vi "mixed-lightsource-velleman.vi"(0 "Power Control":bool, 1 "Shutter VIS":bool, 2 "Shutter UV":bool, 3 "Select NKT System":enum32{"SuperK Varia (VIS)", "Extend-UV"}(radio), 4 "NKT Input Cluster":T2={"Power Level"=5.0, "Feedback Level"=0.0, "Short Wavelength (nm)"=560, "Long Wavelength (nm)"=580, "UV Wavelength (nm)"=400, "Emission On/Off"=FALSE, "Power/Feedback Mode"=FALSE} {"UV Wavelength (nm)" min=350 max=480 step=1; "Long Wavelength (nm)" min=501 max=850 step=1; "Short Wavelength (nm)" min=400 max=560 step=1; "Feedback Level" min=0.0 max=90.0 step=0.1 format="%.1f%%"; "Power Level" min=5.0 max=100.0 step=0.1 format="%.1f%%"}, 5 "Loop Count":i32, 14 "VISA in":refnum<visa-resource-name>, 15 "Init NKT?":bool) -> (6 "Shutter VIS":bool, 7 "Shutter UV 2":bool, 8 "Shutter UV":bool, 9 "Shutter VIS 2":bool, 10 "Laser On!":bool, 11 "Power Control 2":bool, 12 "NKT Output Cluster":T3 {"Feedback Level" format="%.1f%%"; "Power Level" format="%.1f%%"; "Temperature (°C)" format="%.1f"}, 13 "external control input changed?":bool, 17 "long wavelength":T1, 18 "short wavelength":T1, 19 "External Control Input Cluster":T2)   [LabVIEW 2015]
uses:
  <vilib>/Utility/miscctls.llb/LVMinMaxIncTypeDef.ctl
  PLEMv1/K8055D.dll
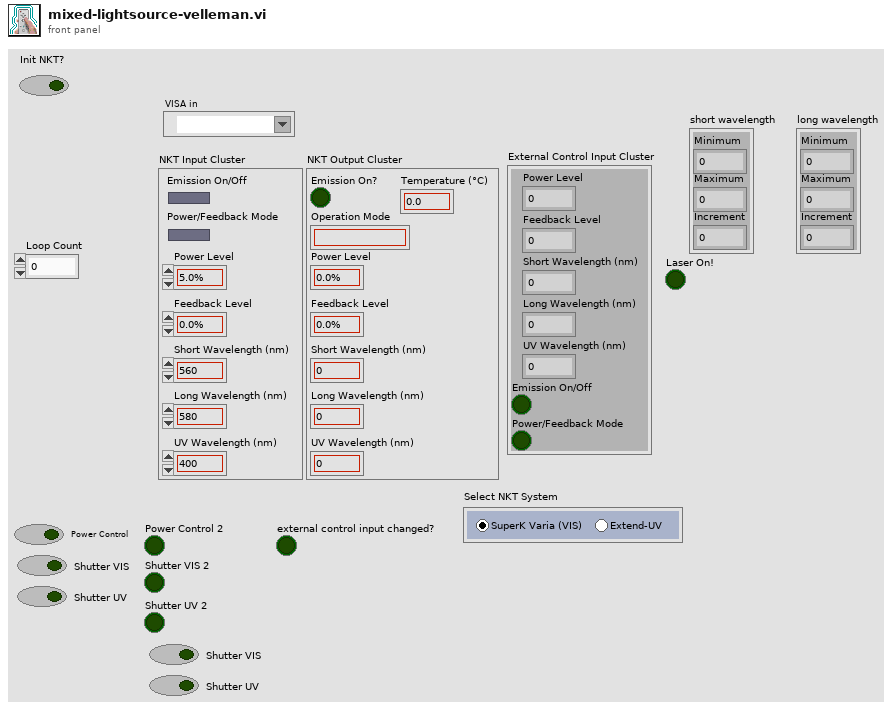
[diagram p1: front panel]
types:
  T1 = typedef "LVMinMaxIncTypeDef.ctl" = cluster{"Minimum":dbl, "Maximum":dbl, "Increment":dbl}
  T2 = cluster{"Power Level":dbl, "Feedback Level":dbl, "Short Wavelength (nm)":i32, "Long Wavelength (nm)":i32, "UV Wavelength (nm)":i32, "Emission On/Off":bool, "Power/Feedback Mode":bool}
  T3 = cluster{"Temperature (°C)":dbl, "Operation Mode":string, "Power Level":dbl, "Feedback Level":dbl, "Short Wavelength (nm)":i32, "Long Wavelength (nm)":i32, "UV Wavelength (nm)":i32, "Emission On?":bool}
  T4 = cluster{"Temperature":dbl, "Operation Mode":string, "Power Level":dbl, "Feedback Level":dbl, "Short Wavelength (nm)":i32, "Long Wavelength (nm)":i32, "UV Wavelength (nm)":i32, "Emission On?":bool}
  T5 = cluster{"Emission On/Off external":bool, "Feedback Level external":dbl, "Power/Feedback Mode external":bool, "Power Level external":dbl}
  T6 = cluster{"Emission On/Off external":bool, "Feedback Level external":bool, "Power/Feedback Mode external":bool, "Power Level external":bool}
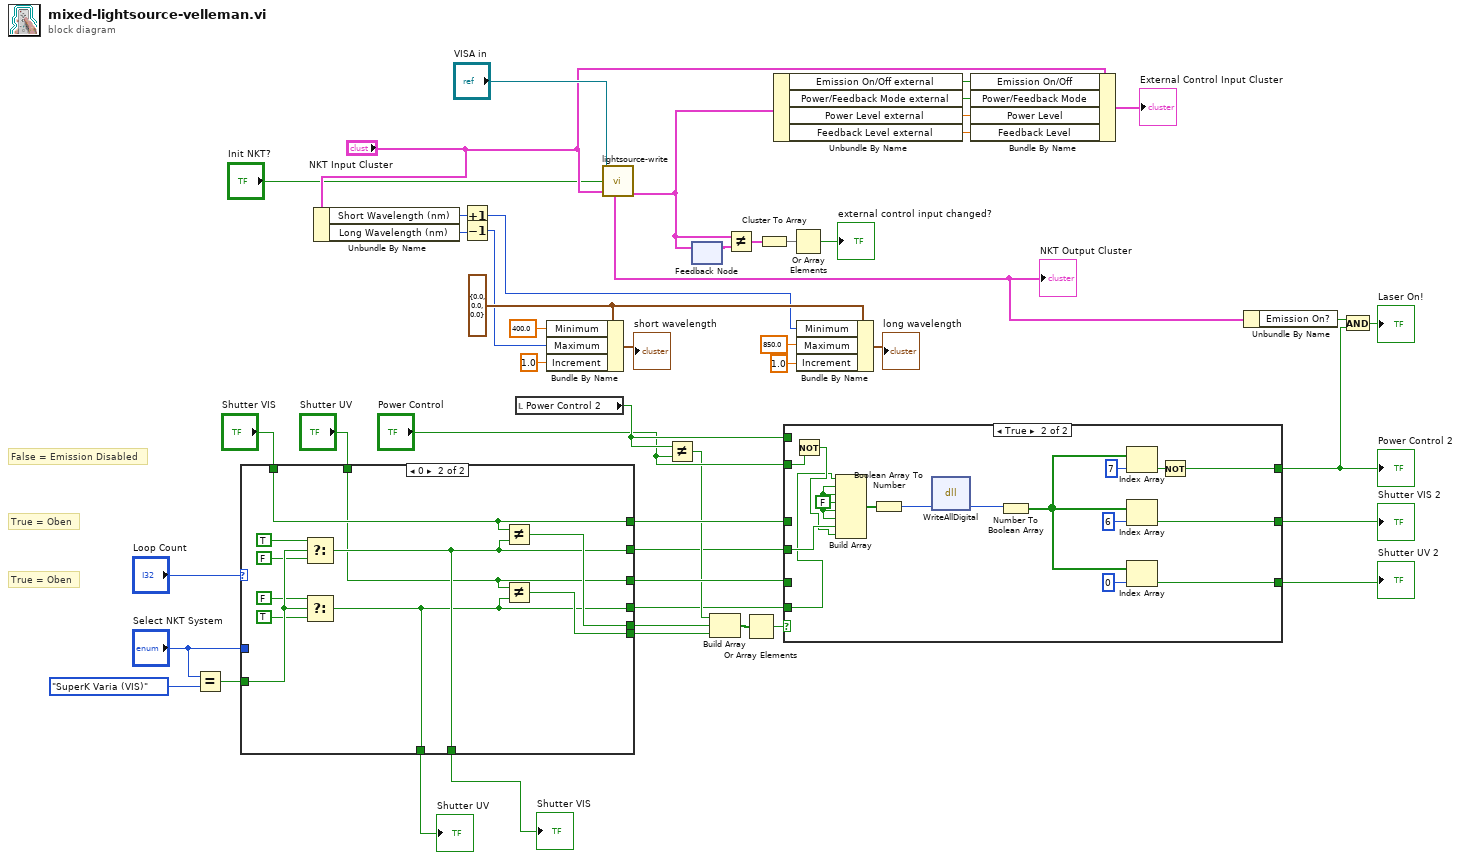
[diagram p0: block diagram]
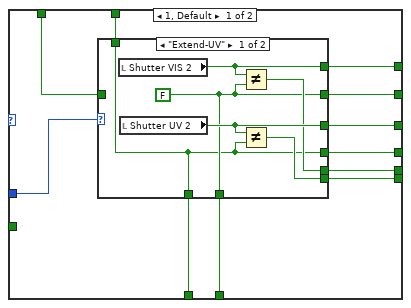
[diagram p2: hidden frame]
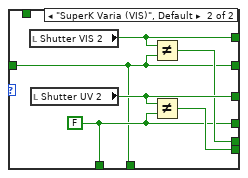
[diagram p3: hidden frame]
diagram:
  w40 = T1 {"Minimum"=0.0, "Maximum"=0.0, "Increment"=0.0} ("Data Entry Limits")
  # "True = Oben"
  # "False = Emission Disabled"
  # "True = Oben"
  n1 = Equal?(x="Select NKT System", y=enum32{"SuperK Varia (VIS)", "Extend-UV"}."SuperK Varia (VIS)" ("Select NKT System")) -> (x = y?=w1:bool)
  n2 = case shown="0" "Loop Count" {
    tunnel: [w60 w74] -> w22
    tunnel: [w59 w73] -> w21
    tunnel: [w58 w83] -> w19
    tunnel: [w57 w82] -> w18
    tunnel: [w56 w81] -> w11
    tunnel: [w55 w80] -> w10
    tunnel: "Select NKT System" -> [w54 _]
    tunnel: [w53 w80] -> w8
    tunnel: [w52 w81] -> w7
    tunnel: "Shutter VIS" -> [w51 w74]
    tunnel: "Shutter UV" -> [w50 w73]
    tunnel: w1 -> [_ w79]
    frame 1, Default {
      n3 = case shown="\"Extend-UV\"" w54 {
        tunnel: [w66 w72] -> w60
        tunnel: [w65 w71] -> w59
        tunnel: [w64 w70] -> w58
        tunnel: [w63 w69] -> w57
        tunnel: [w62 w67] -> w56
        tunnel: [w61 w68] -> w55
        tunnel: [w62 w67] -> w52
        tunnel: [w61 w68] -> w53
        tunnel: w51 -> [_ w67]
        tunnel: w50 -> [w61 _]
        frame "Extend-UV" {
          w62 = FALSE
          n4 = local read "Shutter VIS 2"() -> (w66:bool)
          n5 = local read "Shutter UV 2"() -> (w65:bool)
          n6 = Not Equal?(x=w66, y=w62) -> (x != y?=w64:bool)
          n7 = Not Equal?(x=w65, y=w61) -> (x != y?=w63:bool)
        }
        frame "SuperK Varia (VIS)", Default {
          w68 = FALSE
          n8 = local read "Shutter VIS 2"() -> (w72:bool)
          n9 = local read "Shutter UV 2"() -> (w71:bool)
          n10 = Not Equal?(x=w72, y=w67) -> (x != y?=w70:bool)
          n11 = Not Equal?(x=w71, y=w68) -> (x != y?=w69:bool)
        }
      }
    }
    frame 0 {
      n12 = Select(t=TRUE, s=w79, f=FALSE) -> (s? t:f=w81:bool)
      n13 = Select(t=FALSE, s=w79, f=TRUE) -> (s? t:f=w80:bool)
      n14 = Not Equal?(x=w74, y=w81) -> (x != y?=w83:bool)
      n15 = Not Equal?(x=w73, y=w80) -> (x != y?=w82:bool)
    }
  }
  "Shutter VIS" <- w7
  "Shutter UV" <- w8
  n16 = Unbundle By Name("NKT Input Cluster") -> ("Short Wavelength (nm)"=w38:i32, "Long Wavelength (nm)"=w41:i32)
  n17 = Increment(x=w38) -> (x+1=w37:i32)
  n18 = Decrement(x=w41) -> (x-1=w39:i32)
  n19 = local read "Power Control 2"() -> (w24:bool)
  n20 = Bundle By Name(cluster=w40, "Minimum"=400.0, "Maximum"=w39, "Increment"=1.0) -> (→"short wavelength":T1)
  n21 = call "lightsource-write.vi"("VISA in"="VISA in", "set parameters"="Init NKT?", "NKT Input Cluster"="NKT Input Cluster") -> ("NKT Output Cluster"=w15:T4, "External Control Cluster"=w30:T5)  [unwired: 3 in, 1 out]
  "NKT Output Cluster" <- w15
  n22 = Not Equal?(x=w24, y="Power Control") -> (x != y?=w20:bool)
  n23 = feedback #1() -> (w49:T5)  [unwired: 1 in]
  n24 = feedback-in #1(w30) -> ()
  n25 = Build Array(w20, w19, w18) -> (w17:bool[])
  n26 = Not Equal?(x=w30, y=w49) -> (x != y?=w48:T6)
  n27 = Or Array Elements(Boolean array=w17) -> (logical OR=w16:bool)
  n28 = Cluster To Array(cluster=w48) -> (array=w47:bool[])
  n29 = Unbundle By Name(w30) -> ("Emission On/Off external"=w34:bool, "Power/Feedback Mode external"=w33:bool, "Power Level external"=w32:dbl, "Feedback Level external"=w31:dbl)
  n30 = case shown="True" w16 {
    tunnel: [w85 w97] -> w26
    tunnel: [w84 w94] -> w25
    tunnel: [w86 w92] -> w12
    tunnel: w24 -> [w86 _]
    tunnel: w22 -> [w85 _]
    tunnel: w21 -> [w84 _]
    tunnel: "Power Control" -> [_ w90]
    tunnel: w11 -> [_ w89]
    tunnel: w10 -> [_ w87]
    frame False {
    }
    frame True {
      w102 = FALSE
      n31 = Not(x=w90) -> (.not. x?=w88:bool)
      n32 = Build Array(w87, w102, w102, w102, w102, w102, w89, w88) -> (w101:bool[])
      n33 = Boolean Array To Number(Boolean array=w101) -> (number=w100:u32)
      n34 = dll-call lib="D:/Programs/LabView/playground/PLEMv1/K8055D.dll" fn="WriteAllDigital"(w100) -> (w99:i32)  [unwired: 4 in, 2 out]
      n35 = Number To Boolean Array(number=w99) -> (Boolean array=w93:bool[])
      n36 = Index Array(array=w93, index=7) -> (element=w91:bool)
      n37 = Index Array(array=w93, index=6) -> (element=w97:bool)
      n38 = Index Array(array=w93, index=0) -> (element=w94:bool)
      n39 = Not(x=w91) -> (.not. x?=w92:bool)
    }
  }
  "Power Control 2" <- w12
  "Shutter VIS 2" <- w26
  "Shutter UV 2" <- w25
  n40 = Or Array Elements(Boolean array=w47) -> (logical OR=→"external control input changed?":bool)
  n41 = Bundle By Name(cluster=w40, "Minimum"=w37, "Maximum"=850.0, "Increment"=1.0) -> (→"long wavelength":T1)
  n42 = Bundle By Name(cluster="NKT Input Cluster", "Emission On/Off"=w34, "Power/Feedback Mode"=w33, "Power Level"=w32, "Feedback Level"=w31) -> (→"External Control Input Cluster":T2)
  n43 = Unbundle By Name(w15) -> ("Emission On?"=w13:bool)
  n44 = And(x=w13, y=w12) -> (x .and. y?=→"Laser On!":bool)
